vi "PH_SSAC.Analyse Imgage.vi"(0 "i ref in":refnum<vi>, 5 "error in":errorcluster) -> (14 "i ref out":refnum<vi>, 17 "Status":T1 items=["no info", "off/false/out", "on/true/in", "Failure", "Alarm", "Status 1", "Status 2", "Status 3"], 19 "error out":errorcluster)   [LabVIEW 2014, in "PH_SSAC.lvlib"]
doc: "This VI calculates the fwhm and so on."
uses:
  PH_SSAC.lvlib
  PH_Basics/PH_StatusHandler/PH_StatusHandler.Status.ctl
  <vilib>/Analysis/NI_AALPro.lvlib
  PH_Basics/PH_Common/PH_Common.lvlib
  <vilib>/vision/NI_Vision_Development_Module.lvlib
  PH_Basics/PH_StatusHandler/PH_StatusHandler.lvlib
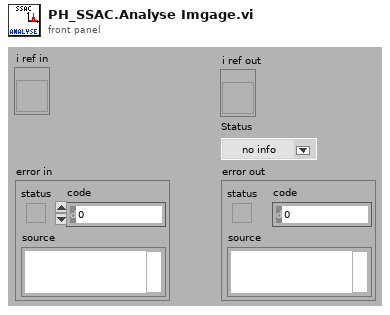
[diagram p1: front panel]
types:
  T1 = typedef "PH_StatusHandler.lvlib/PH_StatusHandler.Status.ctl" = i16
  T2 = typedef "PH_SSAC.lvlib/PH_SSAC.i attribute.ctl" = cluster{"GUI Refs":cluster{"Delete":refnum<vi>, "Global On":refnum<vi>, "Cam Source":refnum<vi>, "Frame Main Signal":refnum<vi>, "Frame Background":refnum<vi>, "dt (Gauss smooth)":refnum<vi>, "Calibration Factor":refnum<vi>, "Background acquire":refnum<vi>, "Threshold":refnum<vi>, "Time evolution of mean pulse duration":refnum<vi>, "Mean Pulse Duration":refnum<vi>, "Main signal":refnum<vi>, "Current Pulse Duration":refnum<vi>, "Processed":refnum<vi>, "Saturation":refnum<vi>, "# for Average":refnum<vi>, "Position":refnum<vi>, "BG Status":refnum<vi>, "Save BG data":refnum<vi>, "Read BG Data":refnum<vi>, "Background Calibration Data":refnum<vi>}, "Images":cluster{"OP Image":T3, "GUI Image":T3, "PSDB Image":T3}, "Global On?":bool, "Frame Main":cluster{"x":u32, "dx":u32, "y":u32, "dy":u32}, "Frame Background":cluster{"x":u32, "dx":u32, "y":u32, "dy":u32}, "dt [fs]":dbl, "Calibration Factor [fs/pixel]":dbl, "Threshold":dbl, "Time evolution of mean pulse duration [fs]":dbl[], "Main Signal":cluster{"Time for Main":dbl[], "Signal":dbl[]}, "Processed":bool, "Current Pulse Duration [fs]":dbl, "# for Average":i32, "Position":i32, "Pulse Durations [fs]":dbl[], "BG":cluster{"Acquire?":bool, "Background Calibration Data":T4, "Save Data":bool}}
  T3 = typedef "IMAQ Image.ctl" = refnum<image>
  T4 = typedef "PH_SSAC.lvlib/PH_SSAC.Background Data.ctl" = cluster{"Date":string, "Time":string, "Frame Main":cluster{"x":u32, "dx":u32, "y":u32, "dy":u32}, "dt [fs]":dbl, "Calibration Factor [fs/pixel]":dbl, "Signal":dbl[], "Frame Background":cluster{"x":u32, "dx":u32, "y":u32, "dy":u32}}
  T5 = typedef "Image Type" = u32
  T6 = cluster{"histogram":u32[], "Minimal Value":sgl, "Maximal Value":sgl, "Starting Value":sgl, "Interval Width":sgl, "Mean Value":sgl, "Standard  Variation":sgl, "Area (pixels)":i32}
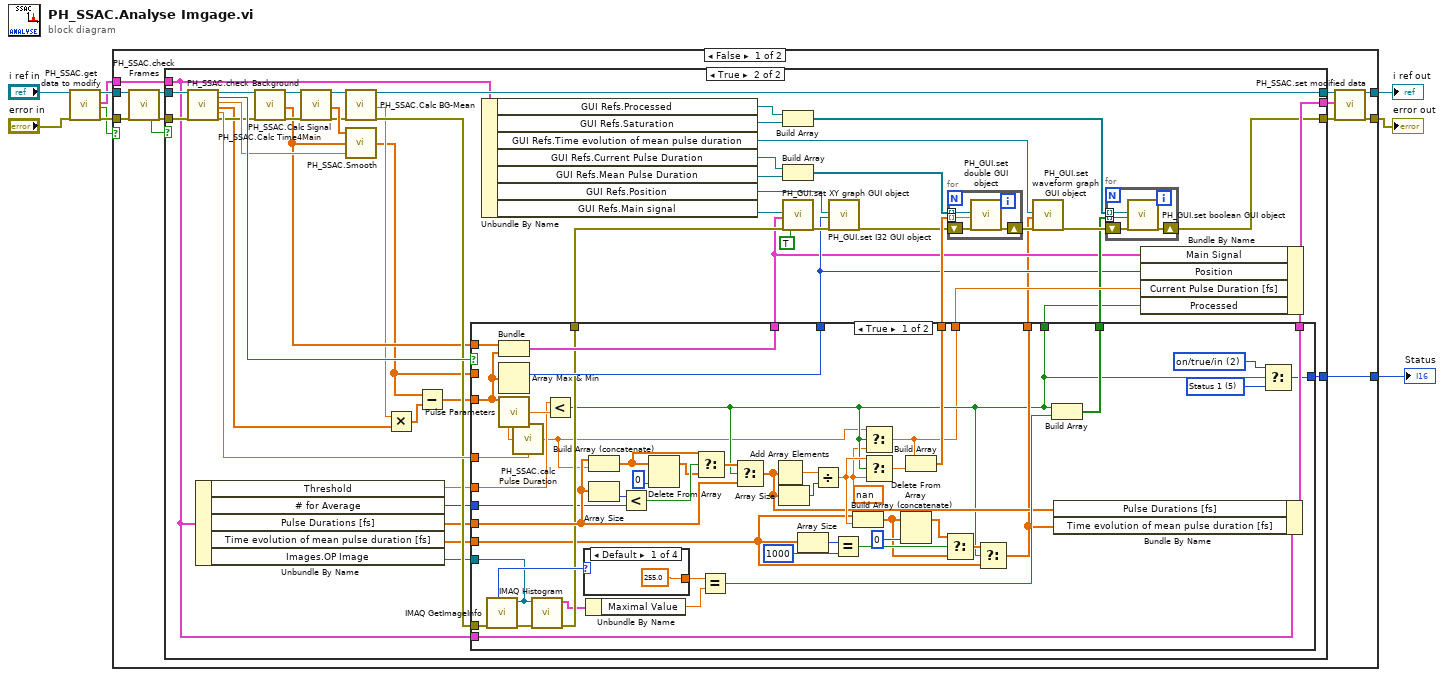
[diagram p0: block diagram]
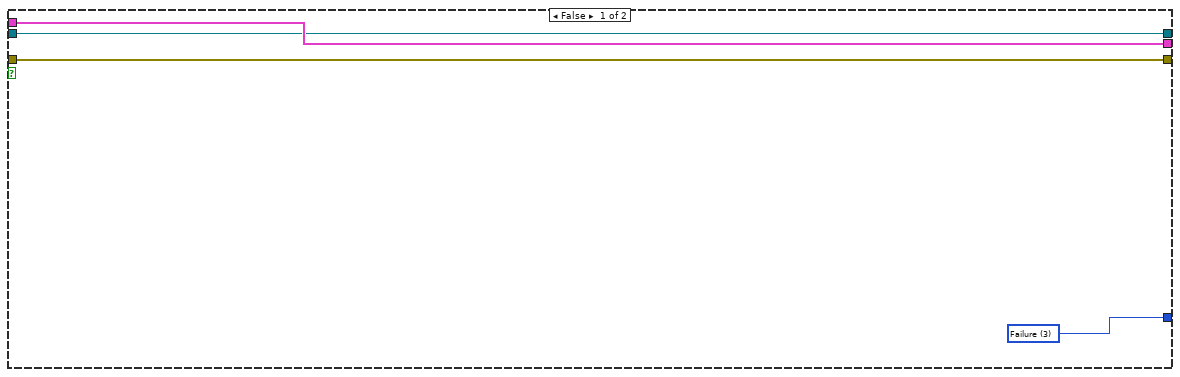
[diagram p2: hidden frame]
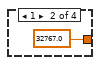
[diagram p3: hidden frame]
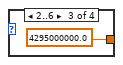
[diagram p4: hidden frame]
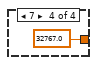
[diagram p5: hidden frame]
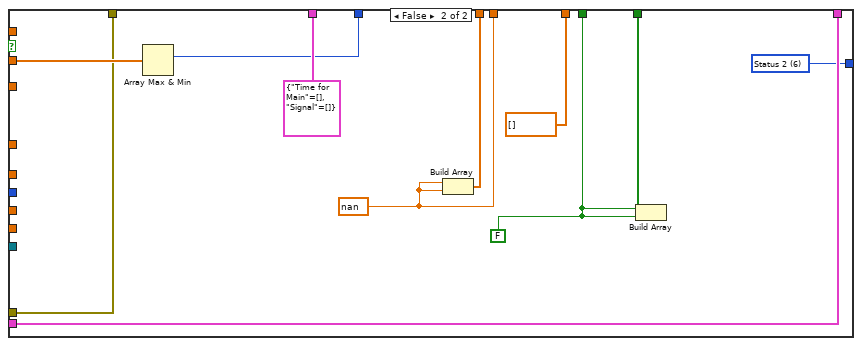
[diagram p6: hidden frame]
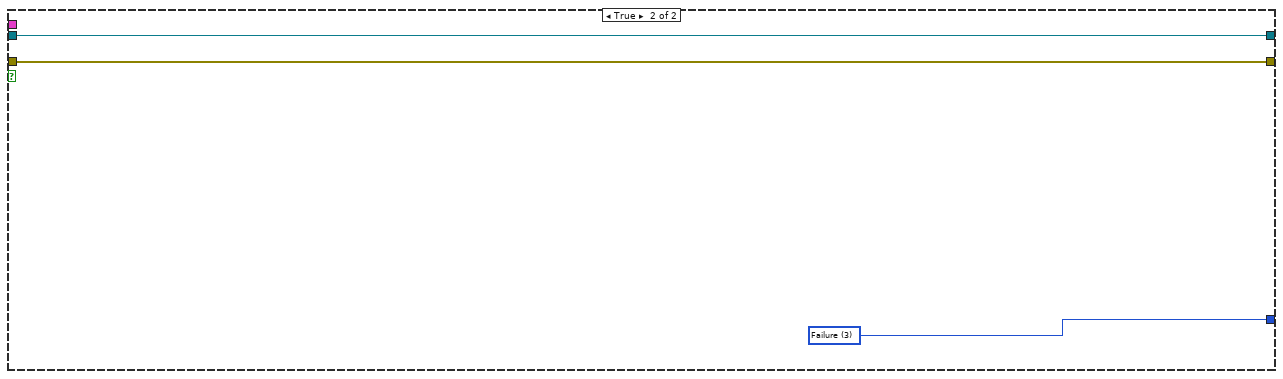
[diagram p7: hidden frame]
diagram:
  n1 = call "PH_SSAC.get data to modify.vi"("i ref in"="i ref in", "error in (no error)"="error in") -> ("i ref out"=w6:refnum<vi>, "i attribute"=w4:T2, "timed out"=w5:bool, "error out"=w7:errorcluster)  [unwired: 14 in]
  n2 = case shown="False" w5 {
    tunnel: w7 -> [w11 w152]
    tunnel: [w21 w152] -> w9
    tunnel: w6 -> [w12 w153]
    tunnel: [w20 w153] -> w8
    tunnel: w4 -> [w17 _]
    tunnel: [w10 w151] -> w1
    frame False {
      n3 = call "PH_SSAC.check Frames.vi"("i ref in"=w12, "error in"=w11) -> ("All ok?"=w13:bool, "i ref out"=w14:refnum<vi>, "error out"=w15:errorcluster)  [unwired: 11 in, 4 out]
      n4 = case shown="True" w13 {
        tunnel: [w25 w73] -> w19
        tunnel: [w23 w50] -> w18
        tunnel: w17 -> [w25 w40]
        tunnel: [w24 w51] -> w16
        tunnel: w15 -> [w23 w76]
        tunnel: w14 -> [w24 w77]
        tunnel: [w22 w26] -> w10
        frame False {
          w22 = T1 3 items=["no info", "off/false/out", "on/true/in", "Failure", "Alarm", "Status 1", "Status 2", "Status 3"] ("f")
        }
        frame True {
          n5 = call "PH_SSAC.check Background.vi"("i ref in"=w77, "error in"=w76) -> ("i ref out"=w52:refnum<vi>, "BG ok?"=w74:bool, "dt [fs]"=w48:dbl, "BG.Background Calibration Data.Signal"=w33:dbl[], "Calibration Factor [fs/pixel]"=w75:dbl, "error out"=w47:errorcluster)  [unwired: 12 in]
          n6 = Unbundle By Name(w40) -> ("Threshold"=w39:dbl, "# for Average"=w34:i32, "Pulse Durations [fs]"=w38:dbl[], "Time evolution of mean pulse duration [fs]"=w37:dbl[], "Images.OP Image"=w36:T3)
          n7 = call "PH_SSAC.Calc Time4Main.vi"("i ref in"=w52, "error in"=w47) -> ("i ref out"=w66:refnum<vi>, "Time for Main [fs]"=w45:dbl[], "error out"=w67:errorcluster)  [unwired: 15 in]
          n8 = call "PH_SSAC.Calc Signal.vi"("i ref in"=w66, "error in"=w67) -> ("i ref out"=w65:refnum<vi>, "Main Frame Linear Averages [pixel]"=w70:dbl[], "error out"=w68:errorcluster)  [unwired: 15 in]
          n9 = call "PH_SSAC.Calc BG-Mean.vi"("i ref in"=w65, "error out"=w68) -> ("i ref out"=w51:refnum<vi>, "BG Mean Value [Pixel]"=w32:dbl, "error out"=w46:errorcluster)  [unwired: 15 in]
          n10 = call "PH_SSAC.Smooth.vi"("dt [fs]"=w48, "Time [fs]"=w45, "Frame Linear Averages [pixel]"=w70) -> ("Signal*Smooth"=w31:dbl[])
          n11 = Multiply(x=w32, y=w33) -> (x*y=w30:dbl[])
          n12 = Subtract(x=w31, y=w30) -> (x-y=w29:dbl[])
          n13 = case shown="True" w74 {
            tunnel: [w134 w150] -> w72
            tunnel: w40 -> [w111 w150]
            tunnel: w75 -> [w121 _]
            tunnel: [w89 w149] -> w35
            tunnel: [w86 w141] -> w71
            tunnel: [w107 w147] -> w49
            tunnel: w31 -> [_ w148]
            tunnel: w46 -> [w120 w147]
            tunnel: w45 -> [w119 _]
            tunnel: [w118 cluster{"Time for Main":dbl[], "Signal":dbl[]} {"Time for Main"=[], "Signal"=[]} ("Main Signal")] -> w41
            tunnel: [w117 w145] -> w42
            tunnel: [w115 w144] -> w44
            tunnel: [w114 dbl[] [] ("Values")] -> w27
            tunnel: [w113 w142] -> w43
            tunnel: w39 -> [w112 _]
            tunnel: w38 -> [w109 _]
            tunnel: w37 -> [w96 _]
            tunnel: w36 -> [w99 _]
            tunnel: w34 -> [w105 _]
            tunnel: w29 -> [w104 _]
            tunnel: [w103 w140] -> w26
            frame True {
              w101 = T1 5 items=["no info", "off/false/out", "on/true/in", "Failure", "Alarm", "Status 1", "Status 2", "Status 3"] ("f")
              w102 = T1 2 items=["no info", "off/false/out", "on/true/in", "Failure", "Alarm", "Status 1", "Status 2", "Status 3"] ("Status")
              w88 = nan ("f")
              n14 = call "IMAQ GetImageInfo"("error in (no error)"=w120, "Image"=w99) -> ("error out"=w100:errorcluster, "Image Type"=w122:T5)  [unwired: 2 in, 6 out]
              n15 = Bundle("Time for Main [fs]"=w119, w104) -> (w118:cluster{"Time for Main [fs]":dbl[], dbl[]})  [unwired: 1 in]
              n16 = Array Max & Min(array=w104) -> (max index (indices)=w117:i32)  [unwired: 3 out]
              n17 = call <vilib>:"Pulse Parameters.vi"("X"=w104) -> ("amplitude"=w135:dbl, "duration"=w125:dbl)  [unwired: 4 in, 9 out]
              n18 = call "PH_SSAC.calc Pulse Duration.vi"("Peak Duration [pixel]"=w125, "Calibration Factor [fs/pixel]"=w121) -> ("Pulse Duration [fs]"=w87:dbl)
              n19 = call "IMAQ Histogram"("error in (no error)"=w100, "Image"=w99) -> ("error out"=w107:errorcluster, "Histogram Report"=w106:T6)  [unwired: 8 in]
              n20 = Less?(x=w112, y=w135) -> (x < y?=w89:bool)
              n21 = case shown="Default" w122 {
                tunnel: [255.0 ("y") 32767.0 ("y") 4295000000.0 ("y") 32767.0 ("y")] -> w98
                frame Default {
                }
                frame 1 {
                }
                frame 2..6 {
                }
                frame 7 {
                }
              }
              n22 = Unbundle By Name(w106) -> ("Maximal Value"=w97:sgl)
              n23 = Build Array (concatenate)(w109, w87) -> (w130:dbl[])
              n24 = Array Size(array=w109) -> (size(s)=w133:i32)
              n25 = Less?(x=w133, y=w105) -> (x < y?=w132:bool)
              n26 = Delete From Array(array=w130, index=0) -> (array with subset deleted=w129:dbl[])  [unwired: 1 in, 1 out]
              n27 = Select(t=w130, s=w132, f=w129) -> (s? t:f=w131:dbl[])
              n28 = Equal?(x=w98, y=w97) -> (x = y?=w123:bool)
              n29 = Select(t=w131, s=w89, f=w109) -> (s? t:f=w116:dbl[])
              n30 = Add Array Elements(numeric array=w116) -> (sum=w128:dbl)
              n31 = Array Size(array=w116) -> (size(s)=w127:i32)
              n32 = Array Size(array=w96) -> (size(s)=w95:i32)
              n33 = Divide(x=w128, y=w127) -> (x/y=w124:dbl)
              n34 = Equal?(x=w95, y=1000) -> (x = y?=w93:bool)
              n35 = Build Array (concatenate)(w96, w124) -> (w90:dbl[])
              n36 = Select(t=w87, s=w89, f=w88) -> (s? t:f=w86:dbl)
              n37 = Select(t=w124, s=w89, f=w88) -> (s? t:f=w126:dbl)
              n38 = Delete From Array(array=w90, index=0) -> (array with subset deleted=w91:dbl[])  [unwired: 1 in, 1 out]
              n39 = Build Array(w86, w126) -> (w115:dbl[])
              n40 = Select(t=w91, s=w93, f=w90) -> (s? t:f=w92:dbl[])
              n41 = Select(t=w92, s=w89, f=w96) -> (s? t:f=w114:dbl[])
              n42 = Build Array(w89, w123) -> (w113:bool[])
              n43 = Bundle By Name(cluster=w111, "Pulse Durations [fs]"=w116, "Time evolution of mean pulse duration [fs]"=w114) -> (w134:T2)
              n44 = Select(t=w102, s=w89, f=w101) -> (s? t:f=w103:T1)
            }
            frame False {
              w140 = T1 6 items=["no info", "off/false/out", "on/true/in", "Failure", "Alarm", "Status 1", "Status 2", "Status 3"] ("f")
              w149 = FALSE
              w141 = nan ("f")
              n45 = Array Max & Min(array=w148) -> (max index (indices)=w145:i32)  [unwired: 3 out]
              n46 = Build Array(w141, w141) -> (w144:dbl[])
              n47 = Build Array(w149, w149) -> (w142:bool[])
            }
          }
          n48 = Unbundle By Name(w40) -> ("GUI Refs.Processed"=w55:refnum<vi>, "GUI Refs.Saturation"=w54:refnum<vi>, "GUI Refs.Time evolution of mean pulse duration"=w57:refnum<vi>, "GUI Refs.Current Pulse Duration"=w60:refnum<vi>, "GUI Refs.Mean Pulse Duration"=w59:refnum<vi>, "GUI Refs.Position"=w61:refnum<vi>, "GUI Refs.Main signal"=w62:refnum<vi>)
          n49 = Build Array(w55, w54) -> (w56:refnum<vi>[])
          n50 = Build Array(w60, w59) -> (w58:refnum<vi>[])
          n51 = call "PH_GUI.set XY graph GUI object.vi"("XY Graph GUI Ref"=w62, "Value Cluster"=w41, "error in"=w49, "Set Full X-Axis (false)"=TRUE) -> ("error out"=w64:errorcluster)  [unwired: 15 in]
          n52 = call "PH_GUI.set I32 GUI object.vi"("I32 GUI Ref"=w61, "value"=w42, "error in (no error)"=w64) -> ("error out"=w28:errorcluster)  [unwired: 16 in]
          n53 = for {
            tunnel: w58 -> [w84] mode=indexing
            tunnel: [w82] -> _ mode=indexing
            shift-right: [w83] -> w69
            shift-left: w28 -> [w85]
            tunnel: w44 -> [w82] mode=indexing
            n54 = call "PH_GUI.set double GUI object.vi"("GUI object Ref"=w84, "value"=w82, "error in (no error)"=w85) -> ("error out"=w83:errorcluster)  [unwired: 16 in]
          }
          n55 = call "PH_GUI.set waveform graph GUI object.vi"("Graph GUI Ref"=w57, "Values"=w27, "error in"=w69) -> ("error out"=w53:errorcluster)  [unwired: 16 in]
          n56 = for {
            tunnel: w43 -> [w81] mode=indexing
            tunnel: w56 -> [w78] mode=indexing
            shift-right: [w79] -> w50
            shift-left: w53 -> [w80]
            n57 = call "PH_GUI.set boolean GUI object.vi"("Boolean Knob GUI Ref"=w78, "Value"=w81, "error in (no error)"=w80) -> ("error out"=w79:errorcluster)  [unwired: 16 in]
          }
          n58 = Bundle By Name(cluster=w72, "Main Signal"=w41, "Position"=w42, "Current Pulse Duration [fs]"=w71, "Processed"=w35) -> (w73:T2)
        }
      }
      n59 = call "PH_SSAC.set modified data.vi"("i ref in"=w16, "i attribute"=w19, "error in (no error)"=w18) -> ("i ref out"=w20:refnum<vi>, "error out"=w21:errorcluster)  [unwired: 15 in]
    }
    frame True {
      w151 = T1 3 items=["no info", "off/false/out", "on/true/in", "Failure", "Alarm", "Status 1", "Status 2", "Status 3"] ("f")
    }
  }
  "error out" <- w9
  "i ref out" <- w8
  "Status" <- w1
